vi "Generate Report.vi"(8 "error in (no error)":errorcluster, 11 "XML Report In":refnum<class "XML Report.lvclass">) -> (0 "error out":errorcluster, 3 "XML Report Out":refnum<class "XML Report.lvclass">)   [LabVIEW 2020, in "Reports.lvlib" / "XML Report.lvclass"]
uses:
  XML Report.lvclass
  Suite Result.ctl
  XML Report.lvclass/XML Report.ctl
  <vilib>/Utility/miscctls.llb/LVMapReplaceAction.ctl
  Core/Result/Status.ctl
  Core/Result/Result.lvlib
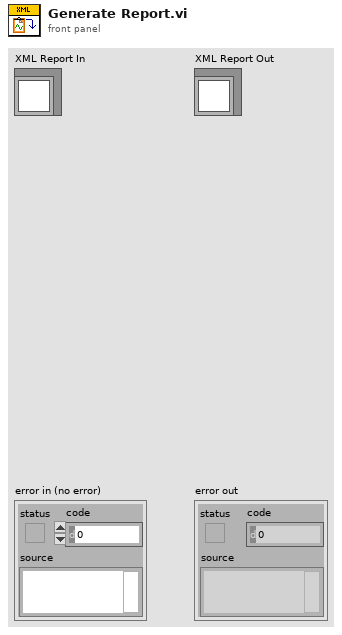
[diagram p1: front panel]
types:
  T1 = typedef "Reports.lvlib/XML Report.lvclass/Suite Result.ctl" = cluster{"Name":string, "Tests":i32, "Failures":i32, "Execution Time":dbl}
  T2 = typedef "Reports.lvlib/XML Report.lvclass/Case Result.ctl" = cluster{"Name":string, "Assertions":i32, "Classname":string, "Status":T3, "Time":dbl}
  T3 = typedef "Result.lvlib/Status.ctl" = enum16{"", "Passed", "Failed", "Error", "Skipped", "Setup Error", "Broken", "Teardown Error"}
  T4 = typedef "LVMapReplaceAction.ctl" = enum32{"Modify Entry only if found", "Add or Modify Entry", "Delete Entry"}
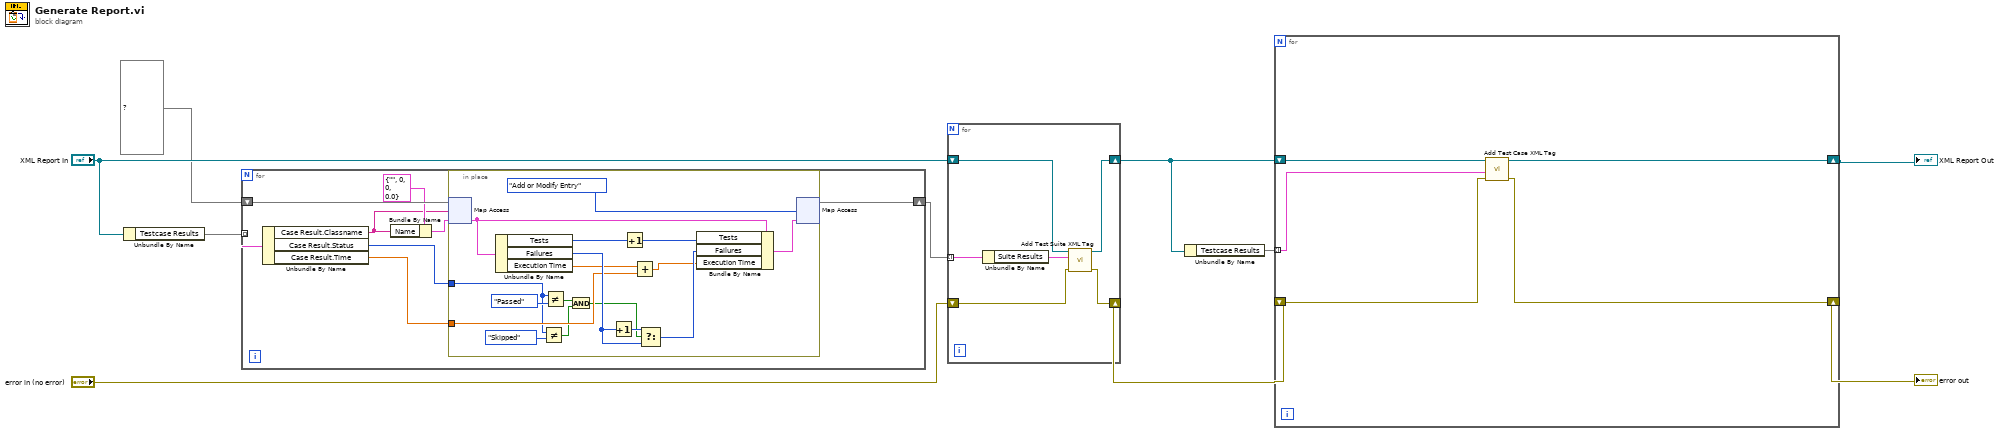
[diagram p0: block diagram]
diagram:
  n1 = Unbundle By Name("XML Report In") -> ("Testcase Results"=w3:map{string, T2})
  n2 = for {
    tunnel: w3 -> [w18] mode=indexing
    shift-right: [w17] -> w2
    shift-left: map{string, T1} {} ("map") -> [w16]
    n3 = Unbundle By Name(w18) -> ("Case Result.Classname"=w14:string, "Case Result.Status"=w12:T3, "Case Result.Time"=w11:dbl)
    n4 = Bundle By Name(cluster=T1 {"Name"="", "Tests"=0, "Failures"=0, "Execution Time"=0.0} ("value"), "Name"=w14) -> (w13:T1)
    n5 = in-place {
      in-place-border: w12 -> [w21]
      in-place-border: w11 -> [w25]
      n6 = in-place-map #1(w16, w14, w13) -> (w34:T1)  [unwired: 1 out]
      n7 = Unbundle By Name(w34) -> ("Tests"=w32:i32, "Failures"=w29:i32, "Execution Time"=w27:dbl)
      n8 = Not Equal?(x=w21, y=Status."Skipped" ("Status")) -> (x != y?=w20:bool)
      n9 = Not Equal?(x=w21, y=Status."Passed" ("Status")) -> (x != y?=w23:bool)
      n10 = And(x=w23, y=w20) -> (x .and. y?=w19:bool)
      n11 = Increment(x=w29) -> (x+1=w30:i32)
      n12 = Increment(x=w32) -> (x+1=w31:i32)
      n13 = Add(x=w27, y=w25) -> (x+y=w26:dbl)
      n14 = Select(t=w30, s=w19, f=w29) -> (s? t:f=w28:i32)
      n15 = Bundle By Name(cluster=w34, "Tests"=w31, "Failures"=w28, "Execution Time"=w26) -> (w33:T1)
      n16 = in-place-map #1(w33, LVMapReplaceAction."Add or Modify Entry" ("action")) -> (w17:map{string, T1})  [unwired: 2 out]
    }
  }
  n17 = for {
    shift-right: [w39] -> w8
    shift-left: "error in (no error)" -> [w40]
    shift-right: [w41] -> w10
    shift-left: "XML Report In" -> [w38]
    tunnel: w2 -> [w37] mode=indexing
    n18 = Unbundle By Name(w37) -> ("Suite Results"=w36:T1)
    n19 = call "Add Test Suite XML Tag.vi"("error in (no error)"=w40, "Suite Results"=w36, "Reports.lvlib:XML Report.lvclass"=w38) -> ("error out"=w39:errorcluster, "output cluster"=w41:refnum<class "XML Report.lvclass">)  [unwired: 7 in]
  }
  n20 = Unbundle By Name(w10) -> ("Testcase Results"=w5:map{string, T2})
  n21 = for {
    shift-right: [w43] -> w6
    shift-left: w8 -> [w44]
    shift-right: [w45] -> w7
    shift-left: w10 -> [w46]
    tunnel: w5 -> [w42] mode=indexing
    n22 = call "Add Test Case XML Tag.vi"("error in (no error)"=w44, "Test Case Result"=w42, "Reports.lvlib:XML Report.lvclass"=w46) -> ("error out"=w43:errorcluster, "output cluster"=w45:refnum<class "XML Report.lvclass">)  [unwired: 7 in]
  }
  "error out" <- w6
  "XML Report Out" <- w7
